vi "SetFocus.vi"(10 "Current \nPosition":dbl[](array[numeric])=[17.0, 17.0, 8.0]) -> (1 "Aborted?":bool, 2 "Destination":dbl[](array[numeric])=[17.0, 17.0, 8.0])   [LabVIEW 2013]
panel:
  in  "Apply":bool
  in  "Cancel":bool
  in  "Run":bool
  in  "Angle to Normal":dbl=60.0
  in  "KinfeThickness":dbl caption="Kinfe Edge Total Thickness"
  in  "FocusPos.":dbl=8.25
  in  "SampleThickness":dbl caption="Sample Total Thickness"
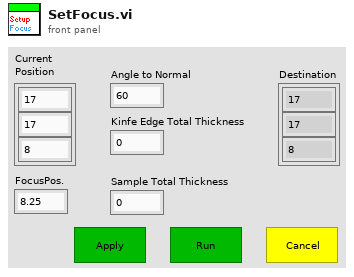
[diagram p1: front panel]
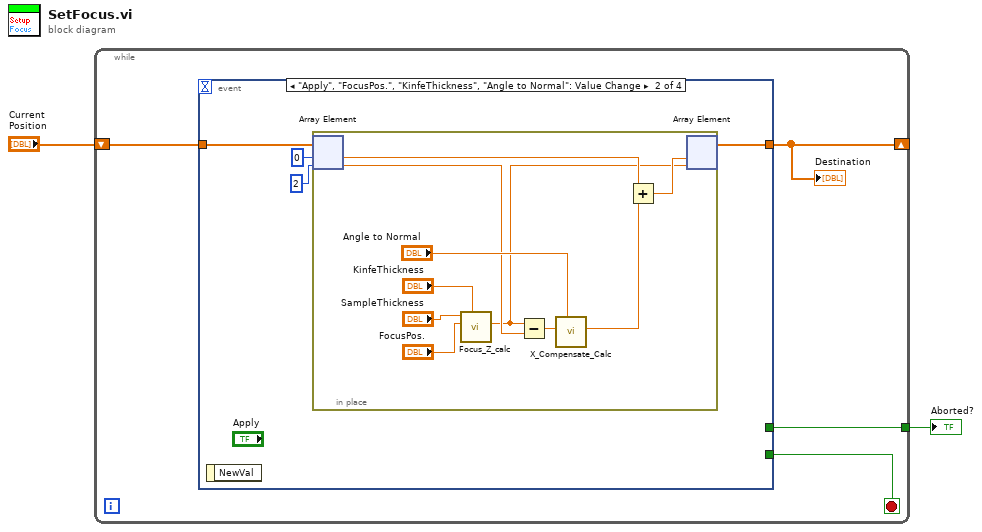
[diagram p0: block diagram]
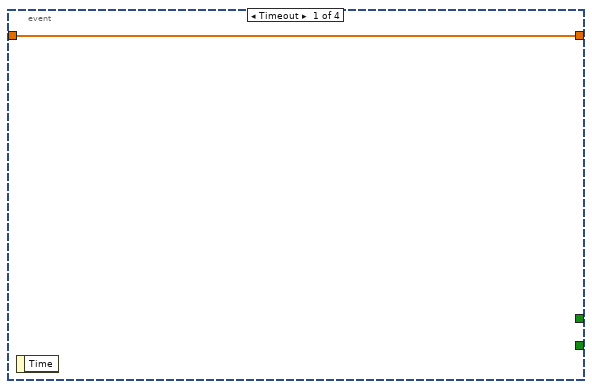
[diagram p2: hidden frame]
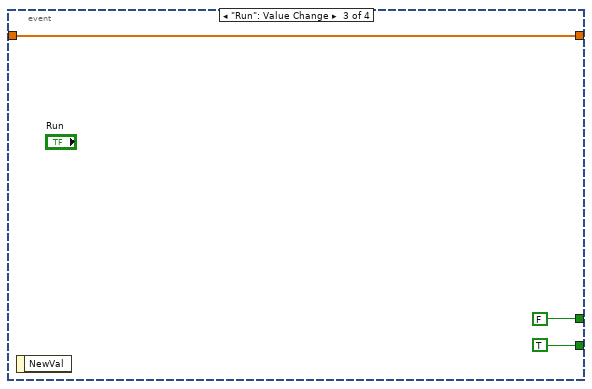
[diagram p3: hidden frame]
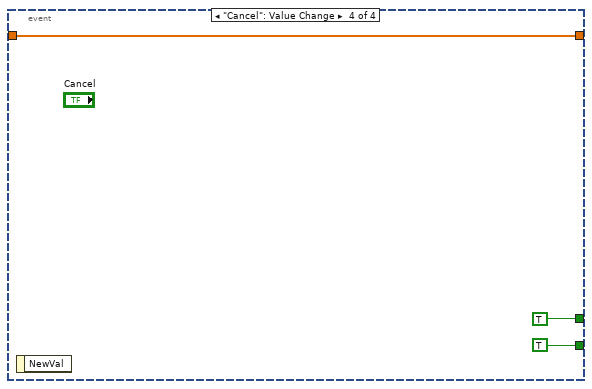
[diagram p4: hidden frame]
diagram:
  n1 = while {
    shift-right: [w5] -> _
    shift-left: "Current \nPosition" -> [w6]
    tunnel: [w3] -> w1
    stop <- w4 stop-if-true
    n2 = event shown="[1] \"Apply\", \"FocusPos.\", \"KinfeThickness\", \"Angle to Normal\": Value Change" {
      selector: _ -> [_ _ _ _]
      dyn-events: _ -> [_ _ _ _]
      timeout: _ -> [_ _ _ _]
      tunnel: w6 -> [w7 w11 w24 w27]
      tunnel: [w7 w10 w24 w27] -> w5
      tunnel: [_ _ TRUE TRUE] -> w4
      tunnel: [_ _ FALSE TRUE] -> w3
      event Timeout {
        n3 = event-data() -> ()  [unwired: 1 in, 1 out]
      }
      event "Apply", "FocusPos.", "KinfeThickness", "Angle to Normal": Value Change {
        n4 = event-data() -> ()  [unwired: 1 in, 1 out]
        n5 = in-place {
          n6 = in-place-array #1(w11, 0, 2) -> (w15:dbl, w13:dbl)
          n7 = call "Focus_Z_calc.vi"("KinfeThickness"="KinfeThickness", "FocusPos."="FocusPos.", "SampleThickness"="SampleThickness") -> ("Z"=w12:dbl)  [unwired: 8 in]
          n8 = Subtract(x=w12, y=w13) -> (x-y=w20:dbl)
          n9 = call "X_Compensate_Calc.vi"("Angle to Normal"="Angle to Normal", "Delta_Z"=w20) -> ("Delta_X"=w14:dbl)  [unwired: 9 in]
          n10 = Add(x=w15, y=w14) -> (x+y=w16:dbl)
          n11 = in-place-array #1(w16, w12) -> (w10:dbl[])  [unwired: 2 out]
        }
      }
      event "Run": Value Change {
        n12 = event-data() -> ()  [unwired: 1 in, 1 out]
      }
      event "Cancel": Value Change {
        n13 = event-data() -> ()  [unwired: 1 in, 1 out]
      }
    }
    "Destination" <- w5
  }
  "Aborted?" <- w1
